vi "Send_lamp_power_supply_command.vi"(10 "write buffer":string="START", 11 "VISA resource name":refnum<visa-resource-name>="COM4") -> ()   [LabVIEW 2016]
uses:
  <vilib>/Instr/_visa.llb/VISA Configure Serial Port (Instr).vi
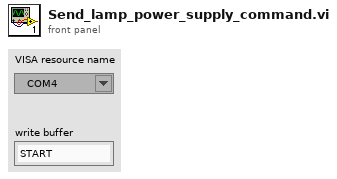
[diagram p1: front panel]
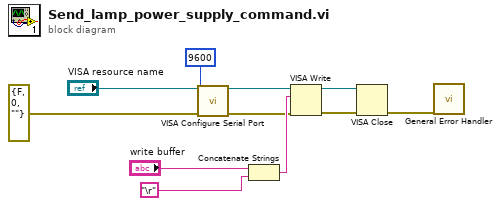
[diagram p0: block diagram]
diagram:
  n1 = call-poly "VISA Configure Serial Port"("VISA resource name"="VISA resource name", "baud rate (9600)"=u32 9600, "error in (no error)"=errorcluster {"status"=FALSE, "code"=0, "source"=""}) -> ("VISA resource name out"=w9:refnum<visa-resource-name>, "error out"=w4:errorcluster)  [unwired: 11 in]
  n2 = Concatenate Strings("write buffer", "\r") -> (w6:string)
  n3 = VISA Write(VISA resource name=w9, write buffer=w6, error in (no error)=w4) -> (VISA resource name out=w5:refnum<visa-resource-name>, error out=w3:errorcluster)  [unwired: 1 out]
  n4 = VISA Close(VISA resource name=w5, error in (no error)=w3) -> (error out=w1:errorcluster)
  n5 = call <vilib>:"General Error Handler.vi"("error in (no error)"=w1) -> ()  [unwired: 10 in, 5 out]
